vi "Add Folder Recursively.vi"(8 "error in (no error)":errorcluster, 9 "Continue Recursing on Error? (F)":bool, 10 "Folder":path, 11 "Session in":refnum<class "Session.lvclass">) -> (0 "error out":errorcluster, 3 "Session out":refnum<class "Session.lvclass">)   [LabVIEW 2020, in "Save for Previous Version.lvlib" / "Session.lvclass"]
uses:
  Session.lvclass
  Session.lvclass/Session.ctl
  <vilib>/Utility/lvfile.llb/NI_FileType.lvlib
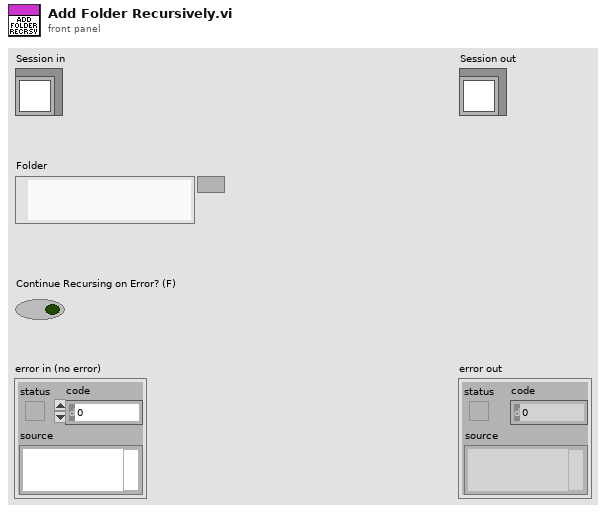
[diagram p1: front panel]
types:
  T1 = typedef "NI_FileType.lvlib/FT_FileTypes.ctl" = enum32{"Invalid file/path", "Unknown type", "Instrument", "Control", "Polymorphic VI", "Project", "Library", "LVClass", "XControl", "XNode", "CIN", "Run-time menu", "Palette menu", "LLB", "Shortcut", "Directory", "Class Private Data Control", "Statechart", "MathScript .m file", "Ladder Diagram", "LVLibp"}
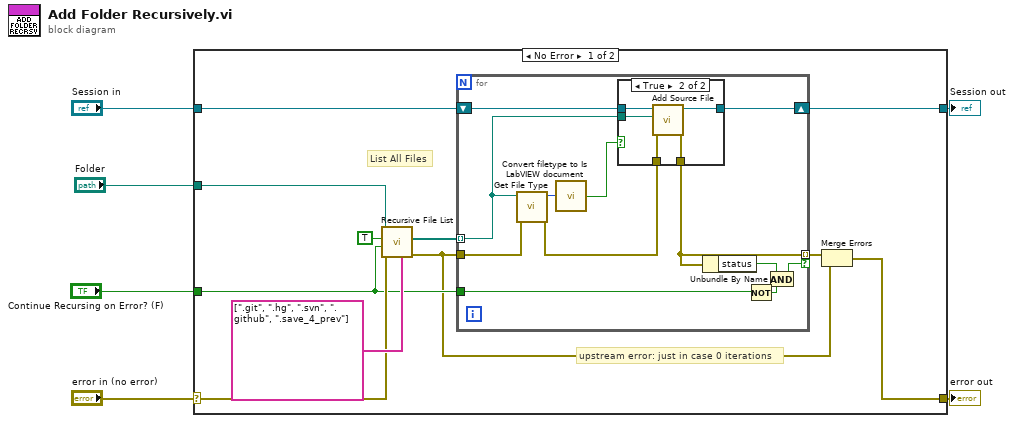
[diagram p0: block diagram]
diagram:
  n1 = case shown="No Error" "error in (no error)" {
    selector: "error in (no error)" -> [w14 w38]
    tunnel: [w8 w38] -> w5
    tunnel: [w11 w37] -> w3
    tunnel: "Session in" -> [w12 w37]
    tunnel: "Folder" -> [w15 _]
    tunnel: "Continue Recursing on Error? (F)" -> [w9 _]
    frame No Error {
      # "upstream error: just in case 0 iterations"
      # "List All Files"
      n2 = call <vilib>:"Recursive File List.vi"("Folders to Exclude"=string[] [".git", ".hg", ".svn", ".github", ".save_4_prev"], "error in (no error)"=w14, "Continue Recursing on Error? (F)"=w9, "Treat LLBs as Folders?"=TRUE, "Folder Path"=w15) -> ("error out"=w7:errorcluster, "All Files in Dir"=w13:path[])  [unwired: 2 in, 3 out]
      n3 = for {
        tunnel: w13 -> [w21] mode=indexing
        tunnel: w7 -> [w18]
        tunnel: [w27] -> w10 mode=indexing if=w23
        tunnel: w9 -> [w26]
        shift-right: [w28] -> w11
        shift-left: w12 -> [w29]
        n4 = call <vilib>:"Get File Type.vi"("error in (no error)"=w18, "path"=w21) -> ("error out"=w19:errorcluster, "file type"=w22:T1)  [unwired: 7 in, 1 out]
        n5 = call <vilib>:"Convert filetype to Is LabVIEW document.vi"("file type"=w22) -> ("Is LabVIEW document?"=w20:bool)  [unwired: 4 in]
        n6 = case shown="True" w20 {
          tunnel: w29 -> [w31 w36]
          tunnel: [w31 w35] -> w28
          tunnel: w19 -> [w30 w34]
          tunnel: [w30 w33] -> w27
          tunnel: w21 -> [_ w32]
          frame False {
          }
          frame True {
            n7 = call "Add Source File.vi"("error in (no error)"=w34, "Source File"=w32, "Session in"=w36) -> ("error out"=w33:errorcluster, "Session out"=w35:refnum<class "Session.lvclass">)  [unwired: 7 in]
          }
        }
        n8 = Unbundle By Name(w27) -> ("status"=w25:bool)
        n9 = Not(x=w26) -> (.not. x?=w24:bool)
        n10 = And(x=w25, y=w24) -> (x .and. y?=w23:bool)
      }
      n11 = Merge Errors(w10, w7) -> (w8:errorcluster)
    }
    frame Error {
    }
  }
  "error out" <- w5
  "Session out" <- w3
